vi "XIPIN_Discrete_Fourier_Transform_3_1.vi"   [LabVIEW 2017]
doc: "The Discrete Fourier Transform (DFT) core has been specifically designed to meet the needs of the LTE standard, in terms of point sizes, low latency and resource requirements.\n------------------------------------\n<b>Need License</b> : No"
uses:
  <vilib>/rvi/XilinxIP/XIPIN_XNode/niFpgaXIPIN.xnode
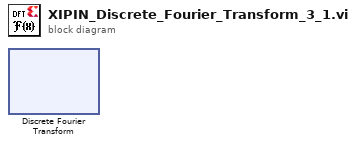
[diagram p0: block diagram]
diagram:
  n1 = xnode ("Discrete Fourier Transform")() -> ()
